vi "LabVIEW-SensorResponseComparison.vi"() -> ()   [LabVIEW 2020]
uses:
  <vilib>/DAQmx/read.llb/DAQmx Read (Analog 2D DBL NChan NSamp).vi
  <vilib>/DAQmx/miscellaneous.llb/DAQmx Fill In Error Info.vi
panel:
  in  "Message Debug Button":bool
  out "Output Waveform Chart":dynamicdata(graph)
  out "LM35 RoC":dbl
  out "Thermistor RoC":dbl
  out "Thermistor Rising":bool
  out "LM35 Rising":bool
  # "Button Off = No message"
  # "Button On = Message"
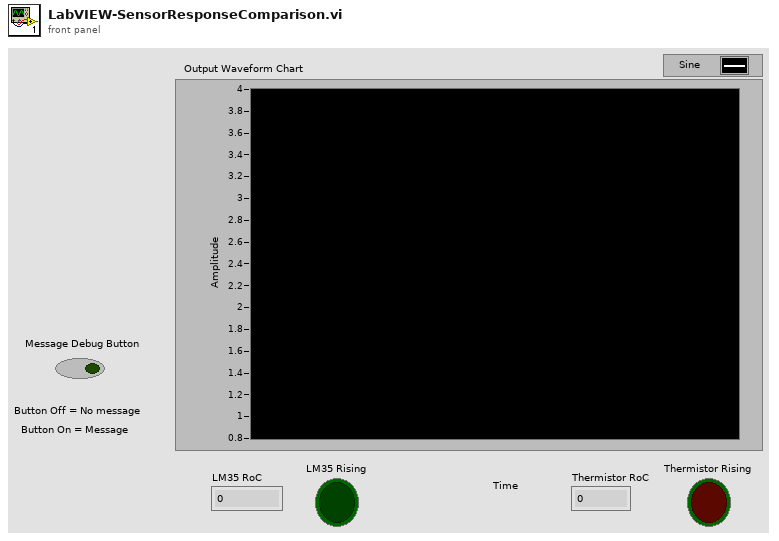
[diagram p1: front panel]
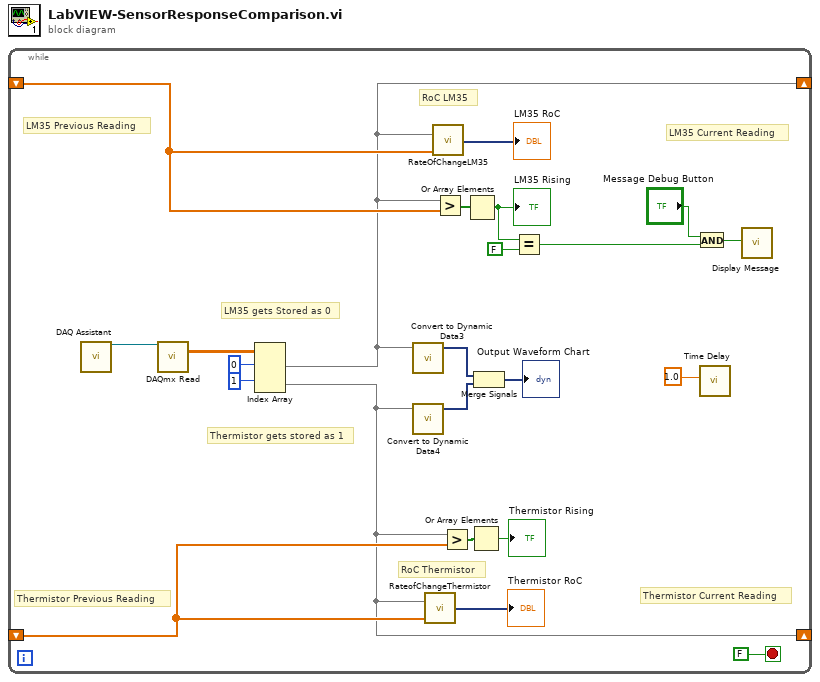
[diagram p0: block diagram]
diagram:
  n1 = while {
    shift-right: [w1] -> _
    shift-left: _ -> [w10]
    shift-right: [w2] -> _
    shift-left: _ -> [w20]
    stop <- FALSE stop-if-true
    # "Thermistor gets stored as 1"
    # "LM35 gets Stored as 0"
    # "Thermistor Current Reading"
    # "Thermistor Previous Reading"
    # "LM35 Previous Reading"
    # "LM35 Current Reading"
    # "RoC Thermistor"
    # "RoC LM35"
    n2 = call "DAQ Assistant"() -> ("task out"=w5:refnum<k21>)  [unwired: 17 in, 2 out]
    n3 = call-poly <vilib>:"DAQmx Read.vi"("task/channels in"=w5) -> ("data"=w6:dbl[][])  [unwired: 12 in, 2 out]
    n4 = Index Array(array=w6, index (row) #1=0 ("index (row)"), index (row) #2=1 ("index (row)")) -> (element #1=w2:dbl[], element #2=w1:dbl[])  [unwired: 2 in]
    n5 = call "Convert to Dynamic Data3"("Array"=w2) -> ("Dynamic Data Type"=w16:dynamicdata)  [unwired: 3 in]
    n6 = call "Convert to Dynamic Data4"("Array"=w1) -> ("Dynamic Data Type"=w15:dynamicdata)  [unwired: 3 in]
    n7 = call "RateofChangeThermistor.vi"("Last Reading"=w10, "Current Reading"=w1) -> ("Rate of Change Output"=→"Thermistor RoC":dynamicdata)  [unwired: 9 in]
    n8 = call "RateOfChangeLM35.vi"("Last Reading"=w20, "Current Reading"=w2) -> ("Rate of Change Output"=→"LM35 RoC":dynamicdata)  [unwired: 9 in]
    n9 = Greater?(x=w2, y=w20) -> (0:w19:bool[])
    n10 = Greater?(x=w1, y=w10) -> (0:w18:bool[])
    n11 = Or Array Elements(Boolean array=w19) -> (logical OR=w12:bool)
    "LM35 Rising" <- w12
    n12 = Or Array Elements(Boolean array=w18) -> (logical OR=→"Thermistor Rising":bool)
    n13 = Merge Signals(w16, w15) -> (→"Output Waveform Chart":dynamicdata)
    n14 = Equal?(x=w12, y=FALSE) -> (x = y?=w7:bool)
    n15 = And(x="Message Debug Button", y=w7) -> (x .and. y?=w8:bool)
    n16 = call "Time Delay"("Delay Time (s)"=1.0) -> ()  [unwired: 10 in, 1 out]
    n17 = call "Display Message"("Enable"=w8) -> ()  [unwired: 9 in, 2 out]
  }
